vi "projectVolume.vi"(0 "input array":u32[][][](array[numeric])) -> (1 "ZY view":u32[][](array[numeric]), 2 "XZ view":u32[][](array[numeric]), 3 "XY view":u32[][](array[numeric]))   [LabVIEW 2010]
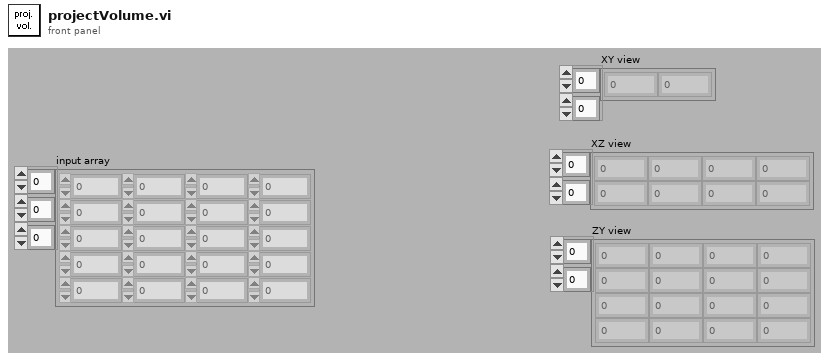
[diagram p1: front panel]
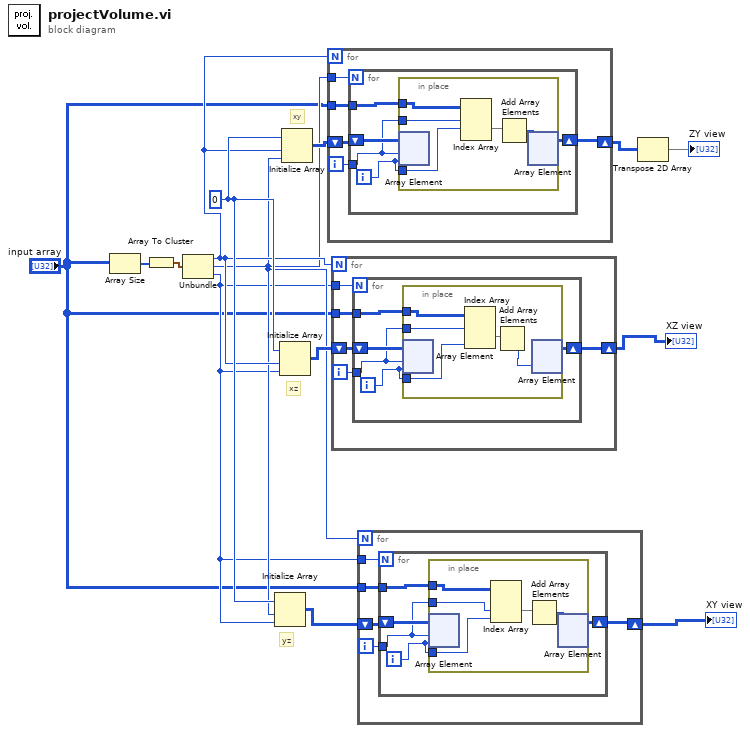
[diagram p0: block diagram]
diagram:
  w11 = u32 0
  # "yz"
  # "xz"
  # "xy"
  n1 = Array Size(array="input array") -> (size(s)=w14:i32[])
  n2 = Array To Cluster(array=w14) -> (cluster=w13:cluster{"[0]":i32, "[1]":i32, "[2]":i32})
  n3 = Unbundle(w13) -> ("[0]"=w10:i32, "[1]"=w8:i32, "[2]"=w7:i32)
  n4 = Initialize Array(w11, w8, w7) -> (w5:u32[][])
  n5 = Initialize Array(w11, w10, w7) -> (w9:u32[][])
  n6 = Initialize Array(w11, w10, w8) -> (w12:u32[][])
  n7 = for {
    N: w10 -> [_]
    tunnel: "input array" -> [w18]
    tunnel: w8 -> [w17]
    shift-right: [w15] -> w4
    shift-left: w12 -> [w19]
    i -> [w16]
    n8 = for {
      N: w17 -> [_]
      tunnel: w18 -> [w23]
      tunnel: w16 -> [w22]
      shift-right: [w20] -> w15
      shift-left: w19 -> [w24]
      i -> [w21]
      n9 = in-place {
        in-place-border: w23 -> [w29]
        in-place-border: w22 -> [w28]
        in-place-border: w21 -> [w26]
        n10 = in-place-array #1(w24, w22, w21) -> ()  [unwired: 1 out]
        n11 = Index Array(array=w29, index (dim 0)=w28, index (dim 1)=w26) -> (element=w27:u32[])  [unwired: 1 in]
        n12 = Add Array Elements(numeric array=w27) -> (sum=w25:u32)
        n13 = in-place-array #1(w25) -> (w20:u32[][])  [unwired: 2 out]
      }
    }
  }
  n14 = for {
    N: w10 -> [_]
    tunnel: "input array" -> [w33]
    tunnel: w7 -> [w32]
    shift-right: [w30] -> w3
    shift-left: w9 -> [w34]
    i -> [w31]
    n15 = for {
      N: w32 -> [_]
      tunnel: w33 -> [w38]
      tunnel: w31 -> [w37]
      shift-right: [w35] -> w30
      shift-left: w34 -> [w39]
      i -> [w36]
      n16 = in-place {
        in-place-border: w38 -> [w44]
        in-place-border: w37 -> [w43]
        in-place-border: w36 -> [w40]
        n17 = in-place-array #2(w39, w37, w36) -> ()  [unwired: 1 out]
        n18 = Index Array(array=w44, index (dim 0)=w43, index (dim 2)=w40) -> (element=w42:u32[])  [unwired: 1 in]
        n19 = Add Array Elements(numeric array=w42) -> (sum=w41:u32)
        n20 = in-place-array #2(w41) -> (w35:u32[][])  [unwired: 2 out]
      }
    }
  }
  "XZ view" <- w3
  n21 = for {
    N: w8 -> [_]
    tunnel: "input array" -> [w48]
    tunnel: w7 -> [w47]
    shift-right: [w45] -> w2
    shift-left: w5 -> [w49]
    i -> [w46]
    n22 = for {
      N: w47 -> [_]
      tunnel: w48 -> [w53]
      tunnel: w46 -> [w52]
      shift-right: [w50] -> w45
      shift-left: w49 -> [w54]
      i -> [w51]
      n23 = in-place {
        in-place-border: w53 -> [w59]
        in-place-border: w52 -> [w55]
        in-place-border: w51 -> [w56]
        n24 = in-place-array #3(w54, w52, w51) -> ()  [unwired: 1 out]
        n25 = Index Array(array=w59, index (dim 1)=w55, index (dim 2)=w56) -> (element=w58:u32[])  [unwired: 1 in]
        n26 = Add Array Elements(numeric array=w58) -> (sum=w57:u32)
        n27 = in-place-array #3(w57) -> (w50:u32[][])  [unwired: 2 out]
      }
    }
  }
  "XY view" <- w2
  n28 = Transpose 2D Array(2D array=w4) -> (transposed array=→"ZY view":u32[][])
